vi "Append Table to Report.vi"   [LabVIEW 2012, in "NI_report.lvclass"]
doc: "Appends a 2D array to a report as a table with the given column width. Wire data to the <B>text data</B> input to determine the polymorphic instance to use or manually select the instance."
uses:
  NI_report.lvclass
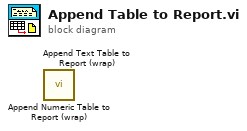
[diagram p0: block diagram]
diagram:
  n1 = call "Append Numeric Table to Report (wrap).vi"() -> ()  [unwired: 12 in, 4 out]
  n2 = call "Append Text Table to Report (wrap).vi"() -> ()  [unwired: 12 in, 4 out]
